vi "State Entry.vi"(8 "error in (no error)":errorcluster, 11 "View Model":T1) -> (0 "error out":errorcluster, 3 "View Model":T1)   [LabVIEW 2017]
doc: "Initializes state information at beginning of transition"
uses:
  View Model/Controls/View Model.ctl
  Error Handler/Controls/Error Model.ctl
  Error Handler/Controls/Error Type.ctl
  View Model/Controls/Shared Model.ctl
  Controls/Elevator Model.ctl
  Controls/Controller Overhead.ctl
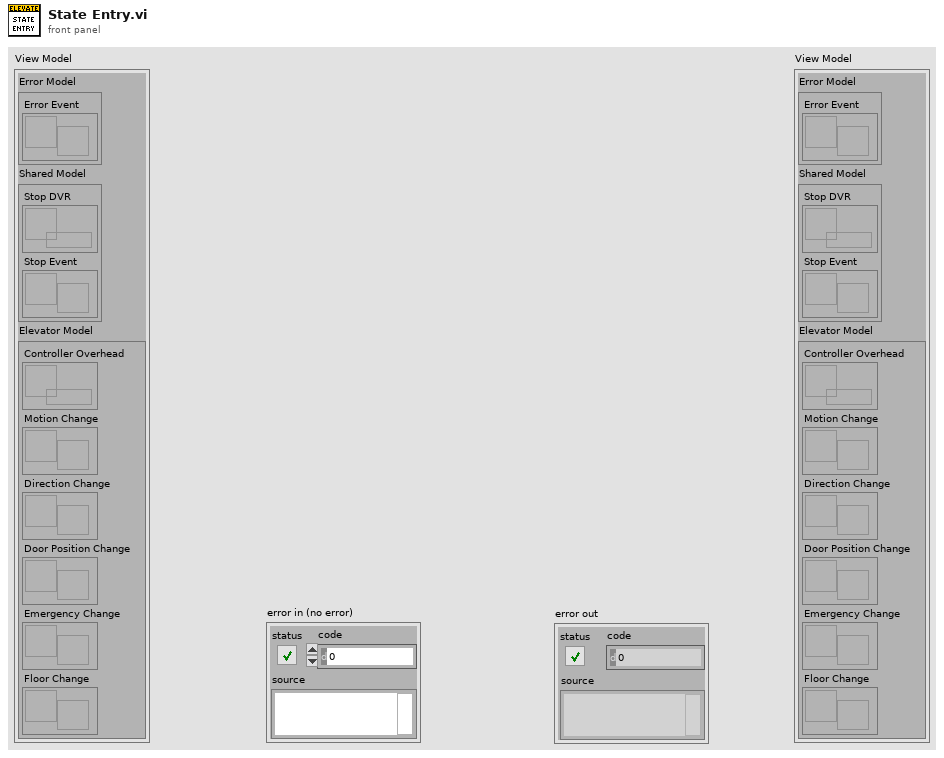
[diagram p1: front panel]
types:
  T1 = typedef "View Model.ctl" = cluster{"Error Model":T2, "Shared Model":T3, "Elevator Model":T4}
  T2 = typedef "Error Model.ctl" = cluster{"Error Event":refnum<user-event>}
  T3 = typedef "Shared Model.ctl" = cluster{"Stop DVR":refnum<data-value>, "Stop Event":refnum<user-event>}
  T4 = typedef "Elevator Model.ctl" = cluster{"Controller Overhead":refnum<data-value>, "Motion Change":refnum<user-event>, "Direction Change":refnum<user-event>, "Door Position Change":refnum<user-event>, "Emergency Change":refnum<user-event>, "Floor Change":refnum<user-event>}
  T5 = enum16{"Idle", "Open Doors", "Close Doors", "Travel", "Emergency"}
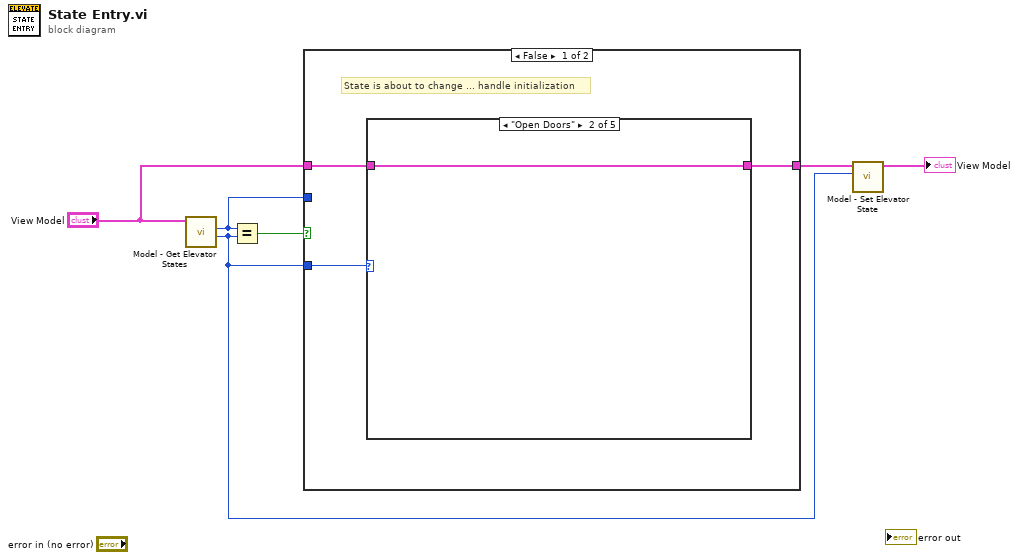
[diagram p0: block diagram]
diagram:
  n1 = call "Model - Get Elevator States.vi"("View Model"="View Model") -> ("Next Elevator State"=w2:T5, "Elevator State"=w5:T5)  [unwired: 7 in, 2 out]
  n2 = Equal?(x=w5, y=w2) -> (x = y?=w6:bool)
  n3 = case shown="False" w6 {
    tunnel: w5 -> [_ _]
    tunnel: w2 -> [w9 _]
    tunnel: "View Model" -> [w8 w15]
    tunnel: [w7 w15] -> w3
    frame False {
      # "State is about to change ... handle initialization"
      n4 = case shown="\"Open Doors\"" w9 {
        tunnel: w8 -> [w10 w11 w12 w13 w14]
        tunnel: [w10 w11 w12 w13 w14] -> w7
        frame "Idle", Default {
        }
        frame "Open Doors" {
        }
        frame "Close Doors" {
        }
        frame "Travel" {
        }
        frame "Emergency" {
        }
      }
    }
    frame True {
    }
  }
  n5 = call "Model - Set Elevator State.vi"("Elevator State"=w2, "View Model"=w3) -> ("View Model"=→"View Model":T1)  [unwired: 8 in, 1 out]
